vi "read exit message.vi"(6 "timeout in ms (1000)":i32=1000, 8 "error in":errorcluster, 11 "data":variant) -> (0 "error out":errorcluster)   [LabVIEW 2015, in "communicator.lvclass"]
uses:
  communicator.lvclass
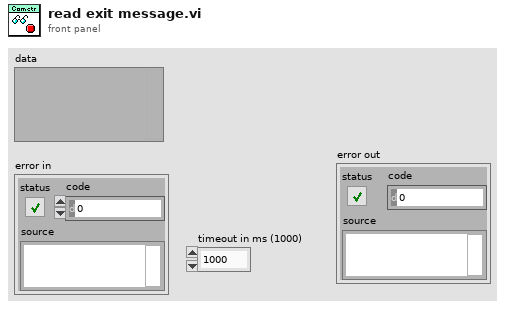
[diagram p1: front panel]
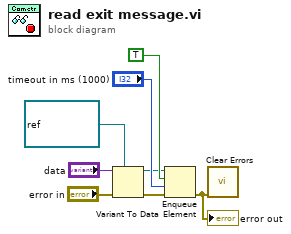
[diagram p0: block diagram]
diagram:
  n1 = Variant To Data(error in="error in", type=refnum<queue> refnum ("queue out"), Variant="data") -> (data=w3:refnum<queue>, error out=w2:errorcluster)
  n2 = Enqueue Element(queue=w3, element=TRUE, timeout in ms (-1)="timeout in ms (1000)", error in (no error)=w2) -> (error out=w1:errorcluster)  [unwired: 2 out]
  "error out" <- w1
  n3 = call <vilib>:"Clear Errors.vi"("error in (no error)"=w1) -> ()  [unwired: 5 in, 2 out]
